vi "Counter.vi"() -> ()   [LabVIEW 2011]
uses:
  <vilib>/DAQmx/write.llb/DAQmx Write (Counter Frequency 1Chan 1Samp).vi
  <vilib>/DAQmx/create/channels.llb/DAQmx Create Channel (CO-Pulse Generation-Frequency).vi
  <vilib>/DAQmx/configure/timing.llb/DAQmx Timing (Implicit).vi
  <vilib>/DAQmx/miscellaneous.llb/DAQmx Fill In Error Info.vi
panel:
  out "Valid Duty Cycle?":bool
  out "coerced(x)":dbl
  in  "counter":tag
  out "error out":errorcluster
  in  "stop":bool
  in  "frequency":dbl=1.0 format="%.6f"
  in  "duty cycle":dbl=0.5 min=0.0 max=1.0 step=0.01 format="%.6f"
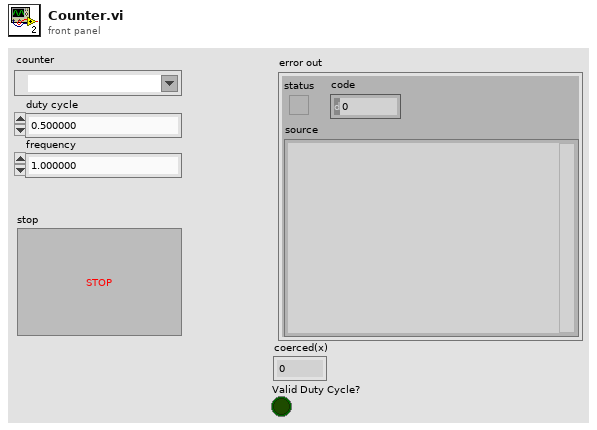
[diagram p1: front panel]
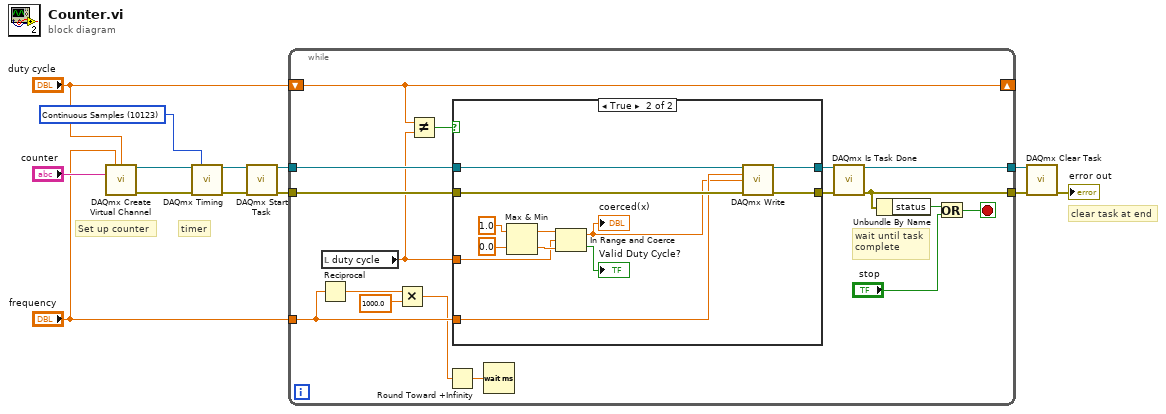
[diagram p0: block diagram]
diagram:
  w11 = 10123 items=["Finite Samples"=10178, "Continuous Samples"=10123, "Hardware Timed Single Point"=12522] ("sample mode")
  # "clear task at end"
  # "timer"
  # "Set up counter"
  n1 = call-poly <vilib>:"DAQmx Create Virtual Channel.vi"("frequency"="frequency", "duty cycle"="duty cycle", "counter"="counter") -> ("task out"=w13:refnum<k21>, "error out"=w12:errorcluster)  [unwired: 11 in]
  n2 = call-poly <vilib>:"DAQmx Timing.vi"("task/channels in"=w13, "sample mode"=w11, "error in"=w12) -> ("task out"=w10:refnum<k21>, "error out"=w9:errorcluster)  [unwired: 11 in]
  n3 = call <vilib>:"DAQmx Start Task.vi"("task/channels in"=w10, "error in"=w9) -> ("task out"=w8:refnum<k21>, "error out"=w7:errorcluster)  [unwired: 12 in]
  n4 = while {
    tunnel: w8 -> [w24]
    tunnel: w7 -> [w23]
    tunnel: [w28] -> w6
    tunnel: [w27] -> w5
    tunnel: "frequency" -> [w18]
    shift-right: [w20] -> _
    shift-left: "duty cycle" -> [w20]
    stop <- w29 stop-if-true
    # "wait until task\ncomplete"
    n5 = Reciprocal(x=w18) -> (1/x=w17:dbl)
    n6 = local read "duty cycle"() -> (w19:dbl)
    n7 = Multiply(x=w17, y=1000.0) -> (x*y=w15:dbl)
    n8 = Not Equal?(x=w20, y=w19) -> (x != y?=w25:bool)
    n9 = Round Toward +Infinity(x=w15) -> (ceil(x): smallest int >= x=w14:dbl)
    n10 = case shown="True" w25 {
      tunnel: w24 -> [w32 w44]
      tunnel: w23 -> [w31 w43]
      tunnel: [w32 w41] -> w22
      tunnel: [w31 w40] -> w21
      tunnel: w18 -> [_ w42]
      tunnel: w19 -> [_ w37]
      frame False {
      }
      frame True {
        n11 = Max & Min(x=1.0, y=0.0) -> (max(x,y)=w38:dbl, min(x,y)=w39:dbl)
        n12 = In Range and Coerce(upper limit=w38, x=w37, lower limit=w39) -> (coerced(x)=w34:dbl, In Range?=→"Valid Duty Cycle?":bool)
        "coerced(x)" <- w34
        n13 = call-poly <vilib>:"DAQmx Write.vi"("task/channels in"=w44, "frequency"=w42, "duty cycle"=w34, "error in"=w43) -> ("task out"=w41:refnum<k21>, "error out"=w40:errorcluster)  [unwired: 9 in, 1 out]
      }
    }
    n14 = Wait (ms)(milliseconds to wait=w14) -> ()  [unwired: 1 out]
    n15 = call <vilib>:"DAQmx Is Task Done.vi"("task/channels in"=w22, "error in"=w21) -> ("task out"=w28:refnum<k21>, "error out"=w27:errorcluster)  [unwired: 11 in, 1 out]
    n16 = Unbundle By Name(w27) -> ("status"=w26:bool)
    n17 = Or(x=w26, y="stop") -> (x .or. y?=w29:bool)
  }
  n18 = call <vilib>:"DAQmx Clear Task.vi"("task in"=w6, "error in"=w5) -> ("error out"=→"error out":errorcluster)  [unwired: 13 in]
